vi "h5_stats.vi"(6 "Attributes":variant, 7 "TYPE":string="STATS_0", 8 "error in (no error)":errorcluster, 9 "statistics":T1, 10 "SQUID":string="1", 11 "H5":path[](array[path])=[path "D:/Data/2015/08/19/20150819_190813/20150819_190813.h5"]) -> (0 "error out":errorcluster, 2 "Exists":bool)   [LabVIEW 2013]
uses:
  Acquisition/statistics.ctl
  <vilib>/addons/h5labview2/file/H5Fmode.ctl
  <vilib>/addons/h5labview2/base/lib_path.vi
  <vilib>/addons/h5labview2/base/H5Equery.vi
  <vilib>/addons/h5labview2/dataset/H5Dwrite.llb/H5Dwrite.xnode
  <vilib>/addons/h5labview2/base/hid_t.ctl
  <vilib>/addons/h5labview2/file/H5F.lvlib
  <vilib>/addons/h5labview2/dataset/H5D.lvlib
  <vilib>/addons/h5labview2/group/H5G.lvlib
  <vilib>/addons/h5labview2/space/H5S.lvlib
  <vilib>/addons/h5labview2/attrib/H5A.lvlib
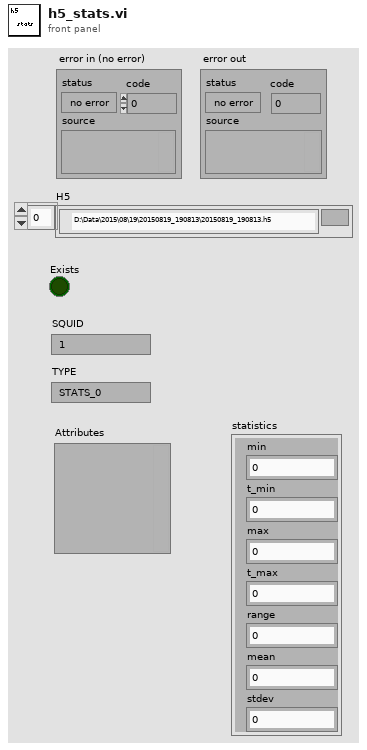
[diagram p1: front panel]
types:
  T1 = typedef "statistics.ctl" = cluster{"min":dbl, "t_min":dbl, "max":dbl, "t_max":dbl, "range":dbl, "mean":dbl, "stdev":dbl}
  T2 = typedef "Semaphore RefNum" = refnum<k1>
  T3 = typedef "H5F.lvlib/H5Fmode.ctl" = enum16{"read-only", "read-write", "overwrite", "create new", "open or create"}
  T4 = typedef "hid_t.ctl" = i32
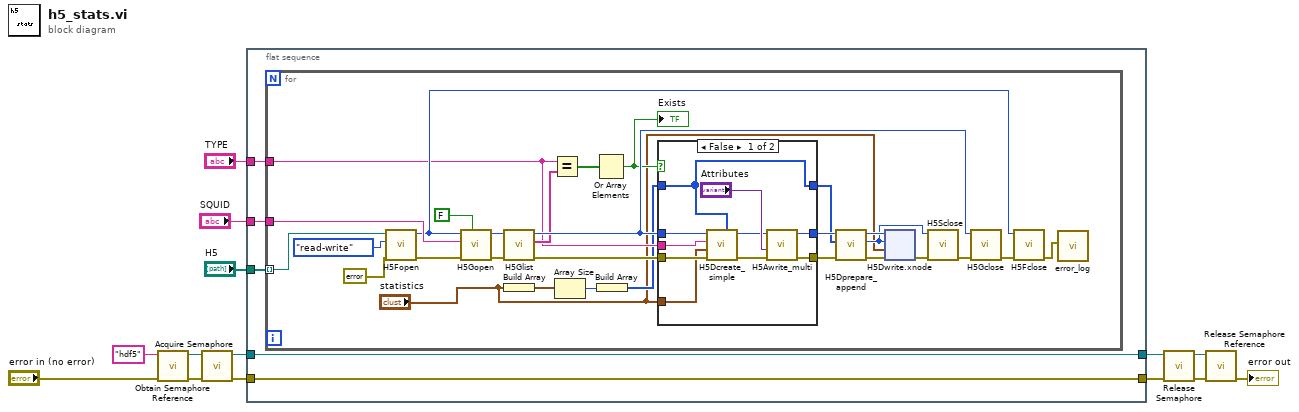
[diagram p0: block diagram]
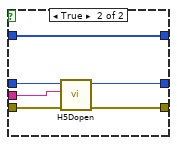
[diagram p2: hidden frame]
diagram:
  n1 = call <vilib>:"Obtain Semaphore Reference.vi"("error in (no error)"="error in (no error)", "name (unnamed)"="hdf5") -> ("error out"=w13:errorcluster, "semaphore"=w14:T2)  [unwired: 3 in, 1 out]
  n2 = call <vilib>:"Acquire Semaphore.vi"("error in (no error)"=w13, "semaphore"=w14) -> ("error out"=w7:errorcluster, "semaphore out"=w6:T2)  [unwired: 3 in, 1 out]
  n3 = flat-sequence {
    tunnel: [w19] -> w8
    tunnel: w7 -> [w19]
    tunnel: w6 -> [w18]
    tunnel: [w18] -> w5
    tunnel: "H5" -> [w17]
    tunnel: "SQUID" -> [w16]
    tunnel: "TYPE" -> [w15]
    frame #0 {
      n4 = for {
        tunnel: w17 -> [w36] mode=indexing
        tunnel: w16 -> [w37]
        tunnel: w15 -> [w28]
        n5 = call <vilib>:"H5Fopen.vi"("error in (no error)"=errorcluster {"status"=FALSE, "code"=0, "source"=""}, "mode (read-only)"=H5Fmode."read-write", "path"=w36) -> ("error out"=w35:errorcluster, "ref out"=w34:T4)  [unwired: 7 in]
        n6 = call <vilib>:"H5Gopen.vi"("create? (F)"=FALSE, "error in (no error)"=w35, "name"=w37, "ref in"=w34) -> ("error out"=w32:errorcluster, "group out"=w33:T4)  [unwired: 6 in]
        n7 = call <vilib>:"H5Glist.vi"("error in (no error)"=w32, "ref in"=w33) -> ("error out"=w31:errorcluster, "names"=w29:string[], "ref out"=w30:T4)  [unwired: 6 in, 1 out]
        n8 = Build Array("statistics") -> (w25:T1[])
        n9 = Equal?(x=w28, y=w29) -> (x = y?=w27:bool[])
        n10 = Array Size(array=w25) -> (size(s)=w24:i32)
        n11 = Or Array Elements(Boolean array=w27) -> (logical OR=w26:bool)
        "Exists" <- w26
        n12 = Build Array(w24) -> (w23:i32[])
        n13 = case shown="False" w26 {
          tunnel: w31 -> [w76 w81]
          tunnel: w30 -> [w75 w78]
          tunnel: w28 -> [w74 w79]
          tunnel: [w71 w80] -> w47
          tunnel: [w72 w77] -> w46
          tunnel: w23 -> [w68 w82]
          tunnel: [w68 w82] -> w43
          tunnel: "statistics" -> [w67 _]
          frame False {
            n14 = call <vilib>:"H5Dcreate_simple.vi"("chunk size"=w68, "error in (no error)"=w76, "type in"=w67, "name"=w74, "ref in"=w75) -> ("error out"=w70:errorcluster, "dset out"=w69:T4)  [unwired: 5 in]
            n15 = call <vilib>:"H5Awrite_multi.vi"("error in (no error)"=w70, "variant in"="Attributes", "ref in"=w69) -> ("error out"=w71:errorcluster, "ref out"=w72:T4)  [unwired: 7 in]
          }
          frame True {
            n16 = call <vilib>:"H5Dopen.vi"("error in (no error)"=w81, "name"=w79, "loc in"=w78) -> ("error out"=w80:errorcluster, "dset out"=w77:T4)  [unwired: 7 in]
          }
        }
        n17 = call <vilib>:"H5Dprepare_append.vi"("error in (no error)"=w47, "append dims"=w43, "dset in"=w46) -> ("error out"=w45:errorcluster, "space out"=w41:T4, "dset out"=w42:T4)  [unwired: 6 in]
        n18 = xnode "H5Dwrite.xnode"("error in (no error)"=w45, "data"="statistics", "file space"=w41, "ref in"=w42) -> ("error out"=w44:errorcluster)  [unwired: 3 in, 2 out]
        n19 = call <vilib>:"H5Sclose.vi"("error in (no error)"=w44, "space in"=w41) -> ("error out"=w40:errorcluster)  [unwired: 9 in]
        n20 = call <vilib>:"H5Gclose.vi"("error in (no error)"=w40, "group in"=w30) -> ("error out"=w38:errorcluster)  [unwired: 9 in]
        n21 = call <vilib>:"H5Fclose.vi"("error in (no error)"=w38, "ref"=w34) -> ("error out"=w21:errorcluster)  [unwired: 9 in]
        n22 = call "error_log.vi"("error"=w21) -> ()  [unwired: 10 in]
      }
    }
  }
  n23 = call <vilib>:"Release Semaphore.vi"("error in (no error)"=w8, "semaphore"=w5) -> ("error out"=w9:errorcluster, "semaphore out"=w10:T2)  [unwired: 4 in]
  n24 = call <vilib>:"Release Semaphore Reference.vi"("error in (no error)"=w9, "semaphore"=w10) -> ("error out"=→"error out":errorcluster)  [unwired: 8 in, 1 out]
